vi "Autonomous Independent.vi"() -> ()   [LabVIEW 2016]
doc: "This VI is called when autonomous begins, and will automatically be terminated when autonomous ends. You can carry out timed or sensor driven robot movement independently without needing to return to the caller."
uses:
  <vilib>/Rock Robotics/Network Tables/NT Read Number.vi
  Global 2.vi
  Systems/Global 1.vi
panel:
  out "Present (s)":dbl=3576005670.903064
  out "Time has Elapsed":bool=TRUE
  out "Elapsed Time (s)":dbl=0.26720476150512695
  out "Gyro":dbl=0.23233298402160002
  in  "Oscillate effort":dbl=0.25 format="%#_13g"
  out "Auto Mode":dbl=13.0
  in  "Auton_Modes":T1(array[cluster])=[{"Actions"=[{"Effort"=0.55, "Duration"=3.5, "Action"=enum."Vision Correction", "Encoder"=0.0, "Condition"=FALSE}, {"Effort"=0.0, "Duration"=0.0, "Action"=enum."Nothing", "Encoder"=0.0, "Condition"=FALSE}]}, {"Actions"=[{"Effort"=0.0, "Duration"=0.1, "Action"=enum."Drive Encoder Reset", "Encoder"=0.0, "Condition"=FALSE}, {"Effort"=0.0, "Duration"=0.1, "Action"=enum."Gyro Reset", "Encoder"=0.0, "Condition"=FALSE}, {"Effort"=0.0, "Duration"=4.0, "Action"=enum."Drive", "Encoder"=62.0, "Condition"=FALSE}, {"Effort"=0.15, "Duration"=0.1, "Action"=enum."Turn", "Encoder"=-55.0, "Condition"=FALSE}, {"Effort"=0.0, "Duration"=0.1, "Action"=enum."Gyro Reset", "Encoder"=0.0, "Condition"=FALSE}, {"Effort"=0.0, "Duration"=0.1, "Action"=enum."Drive Encoder Reset", "Encoder"=0.0, "Condition"=FALSE}, {"Effort"=0.0, "Duration"=4.0, "Action"=enum."Drive", "Encoder"=76.0, "Condition"=FALSE}, {"Effort"=1.0, "Duration"=0.25, "Action"=enum."Gear0", "Encoder"=0.0, "Condition"=FALSE}, {"Effort"=0.0, "Duration"=0.1, "Action"=enum."Drive Encoder Reset", "Encoder"=3.0, "Condition"=FALSE}, {"Effort"=0.0, "Duration"=3.0, "Action"=enum."Drive", "Encoder"=-36.0, "Condition"=FALSE}, {"Effort"=0.08, "Duration"=0.0, "Action"=enum."Turn", "Encoder"=15.5, "Condition"=FALSE}, {"Effort"=0.0, "Duration"=0.1, "Action"=enum."Gyro Reset", "Encoder"=0.0, "Condition"=FALSE}, {"Effort"=0.0, "Duration"=0.5, "Action"=enum."Drive Encoder Reset", "Encoder"=0.0, "Condition"=FALSE}, {"Effort"=0.0, "Duration"=5.0, "Action"=enum."Drive", "Encoder"=-94.0, "Condition"=TRUE}]}, {"Actions"=[{"Effort"=0.0, "Duration"=0.1, "Action"=enum."Drive Encoder Reset", "Encoder"=0.0, "Condition"=FALSE}, {"Effort"=0.0, "Duration"=0.1, "Action"=enum."Gyro Reset", "Encoder"=0.0, "Condition"=FALSE}, {"Effort"=0.0, "Duration"=4.0, "Action"=enum."Drive", "Encoder"=76.0, "Condition"=FALSE}, {"Effort"=1.0, "Duration"=0.5, "Action"=enum."Gear0", "Encoder"=0.0, "Condition"=FALSE}, {"Effort"=1.0, "Duration"=0.0, "Action"=enum."Nothing", "Encoder"=0.0, "Condition"=FALSE}, {"Effort"=1.0, "Duration"=0.0, "Action"=enum."Nothing", "Encoder"=0.0, "Condition"=FALSE}, {"Effort"=0.0, "Duration"=0.0, "Action"=enum."Drive Encoder Reset", "Encoder"=0.0, "Condition"=FALSE}, {"Effort"=0.0, "Duration"=0.0, "Action"=enum."Nothing", "Encoder"=0.0, "Condition"=FALSE}, {"Effort"=0.0, "Duration"=0.0, "Action"=enum."Nothing", "Encoder"=0.0, "Condition"=FALSE}, {"Effort"=0.0, "Duration"=10000.0, "Action"=enum."Drive", "Encoder"=-24.0, "Condition"=FALSE}, {"Effort"=0.0, "Duration"=0.0, "Action"=enum."Drive Encoder Reset", "Encoder"=0.0, "Condition"=FALSE}, {"Effort"=-0.4, "Duration"=5.0, "Action"=enum."Nothing", "Encoder"=70.0, "Condition"=FALSE}]}, {"Actions"=[{"Effort"=0.0, "Duration"=0.1, "Action"=enum."Drive Encoder Reset", "Encoder"=6.462, "Condition"=FALSE}, {"Effort"=0.0, "Duration"=0.1, "Action"=enum."Gyro Reset", "Encoder"=0.0, "Condition"=FALSE}, {"Effort"=0.0, "Duration"=1.0, "Action"=enum."Drive", "Encoder"=60.0, "Condition"=FALSE}, {"Effort"=0.15, "Duration"=0.1, "Action"=enum."Turn", "Encoder"=55.0, "Condition"=FALSE}, {"Effort"=0.0, "Duration"=0.1, "Action"=enum."Gyro Reset", "Encoder"=0.0, "Condition"=FALSE}, {"Effort"=-0.25, "Duration"=0.0, "Action"=enum."Drive Encoder Reset", "Encoder"=7.5, "Condition"=FALSE}, {"Effort"=0.0, "Duration"=4.0, "Action"=enum."Drive", "Encoder"=76.0, "Condition"=FALSE}, {"Effort"=1.0, "Duration"=0.25, "Action"=enum."Gear0", "Encoder"=0.0, "Condition"=FALSE}, {"Effort"=0.0, "Duration"=0.1, "Action"=enum."Drive Encoder Reset", "Encoder"=0.0, "Condition"=FALSE}, {"Effort"=0.0, "Duration"=3.0, "Action"=enum."Drive", "Encoder"=-36.0, "Condition"=FALSE}, {"Effort"=0.08, "Duration"=0.0, "Action"=enum."Turn", "Encoder"=-60.0, "Condition"=FALSE}, {"Effort"=0.0, "Duration"=0.1, "Action"=enum."Gyro Reset", "Encoder"=0.0, "Condition"=FALSE}, {"Effort"=0.0, "Duration"=0.5, "Action"=enum."Drive Encoder Reset", "Encoder"=0.0, "Condition"=FALSE}, {"Effort"=0.0, "Duration"=5.0, "Action"=enum."Drive", "Encoder"=30.0, "Condition"=TRUE}]}, {"Actions"=[{"Effort"=0.0, "Duration"=0.1, "Action"=enum."Drive Encoder Reset", "Encoder"=6.462, "Condition"=FALSE}, {"Effort"=0.0, "Duration"=0.1, "Action"=enum."Gyro Reset", "Encoder"=0.0, "Condition"=FALSE}, {"Effort"=0.0, "Duration"=1.0, "Action"=enum."Drive", "Encoder"=60.0, "Condition"=FALSE}, {"Effort"=0.15, "Duration"=0.1, "Action"=enum."Turn", "Encoder"=-55.0, "Condition"=FALSE}, {"Effort"=0.0, "Duration"=0.1, "Action"=enum."Gyro Reset", "Encoder"=0.0, "Condition"=FALSE}, {"Effort"=-0.25, "Duration"=0.0, "Action"=enum."Drive Encoder Reset", "Encoder"=7.5, "Condition"=FALSE}, {"Effort"=0.0, "Duration"=4.0, "Action"=enum."Drive", "Encoder"=76.0, "Condition"=FALSE}, {"Effort"=1.0, "Duration"=0.25, "Action"=enum."Gear0", "Encoder"=0.0, "Condition"=FALSE}, {"Effort"=0.0, "Duration"=0.1, "Action"=enum."Drive Encoder Reset", "Encoder"=0.0, "Condition"=FALSE}, {"Effort"=0.0, "Duration"=3.0, "Action"=enum."Drive", "Encoder"=-36.0, "Condition"=FALSE}, {"Effort"=0.08, "Duration"=0.0, "Action"=enum."Turn", "Encoder"=60.0, "Condition"=FALSE}, {"Effort"=0.0, "Duration"=0.1, "Action"=enum."Gyro Reset", "Encoder"=0.0, "Condition"=FALSE}, {"Effort"=0.0, "Duration"=0.5, "Action"=enum."Drive Encoder Reset", "Encoder"=0.0, "Condition"=FALSE}, {"Effort"=0.0, "Duration"=5.0, "Action"=enum."Drive", "Encoder"=30.0, "Condition"=TRUE}]}, {"Actions"=[{"Effort"=0.0, "Duration"=0.1, "Action"=enum."Drive Encoder Reset", "Encoder"=0.0, "Condition"=FALSE}, {"Effort"=0.0, "Duration"=0.1, "Action"=enum."Gyro Reset", "Encoder"=0.0, "Condition"=FALSE}, {"Effort"=0.0, "Duration"=4.0, "Action"=enum."Drive", "Encoder"=62.0, "Condition"=FALSE}, {"Effort"=0.15, "Duration"=0.1, "Action"=enum."Turn", "Encoder"=55.0, "Condition"=FALSE}, {"Effort"=0.0, "Duration"=0.1, "Action"=enum."Gyro Reset", "Encoder"=0.0, "Condition"=FALSE}, {"Effort"=0.0, "Duration"=0.1, "Action"=enum."Drive Encoder Reset", "Encoder"=0.0, "Condition"=FALSE}, {"Effort"=0.0, "Duration"=4.0, "Action"=enum."Drive", "Encoder"=76.0, "Condition"=FALSE}, {"Effort"=1.0, "Duration"=0.25, "Action"=enum."Gear0", "Encoder"=0.0, "Condition"=FALSE}, {"Effort"=0.0, "Duration"=0.1, "Action"=enum."Drive Encoder Reset", "Encoder"=3.0, "Condition"=FALSE}, {"Effort"=0.0, "Duration"=3.0, "Action"=enum."Drive", "Encoder"=-36.0, "Condition"=FALSE}, {"Effort"=0.08, "Duration"=0.0, "Action"=enum."Turn", "Encoder"=-15.5, "Condition"=FALSE}, {"Effort"=0.0, "Duration"=0.1, "Action"=enum."Gyro Reset", "Encoder"=0.0, "Condition"=FALSE}, {"Effort"=0.0, "Duration"=0.5, "Action"=enum."Drive Encoder Reset", "Encoder"=0.0, "Condition"=FALSE}, {"Effort"=0.0, "Duration"=5.0, "Action"=enum."Drive", "Encoder"=-94.0, "Condition"=TRUE}]}, {"Actions"=[{"Effort"=0.0, "Duration"=0.1, "Action"=enum."Nothing", "Encoder"=0.0, "Condition"=FALSE}, {"Effort"=0.0, "Duration"=0.1, "Action"=enum."Gyro Reset", "Encoder"=0.0, "Condition"=FALSE}, {"Effort"=0.25, "Duration"=5.0, "Action"=enum."Drive", "Encoder"=60000.0, "Condition"=TRUE}, {"Effort"=0.75, "Duration"=1.0, "Action"=enum."Nothing", "Encoder"=0.0, "Condition"=FALSE}, {"Effort"=0.0, "Duration"=1.0, "Action"=enum."Nothing", "Encoder"=0.0, "Condition"=FALSE}, {"Effort"=0.0, "Duration"=0.0, "Action"=enum."Nothing", "Encoder"=0.0, "Condition"=FALSE}]}, {"Actions"=[{"Effort"=0.0, "Duration"=0.1, "Action"=enum."Drive Encoder Reset", "Encoder"=0.0, "Condition"=FALSE}, {"Effort"=0.0, "Duration"=0.1, "Action"=enum."Gyro Reset", "Encoder"=0.0, "Condition"=FALSE}, {"Effort"=0.3, "Duration"=0.0, "Action"=enum."Drive", "Encoder"=24.0, "Condition"=FALSE}, {"Effort"=0.3, "Duration"=3.0, "Action"=enum."Nothing", "Encoder"=0.0, "Condition"=FALSE}, {"Effort"=0.3, "Duration"=2.0, "Action"=enum."Vision Correction", "Encoder"=30.0, "Condition"=FALSE}, {"Effort"=0.2, "Duration"=1.0, "Action"=enum."Drive", "Encoder"=18.5, "Condition"=TRUE}, {"Effort"=1.0, "Duration"=0.0, "Action"=enum."Gear0", "Encoder"=0.0, "Condition"=FALSE}, {"Effort"=-0.2, "Duration"=1.3, "Action"=enum."Drive", "Encoder"=30.0, "Condition"=TRUE}, {"Effort"=0.0, "Duration"=3.0, "Action"=enum."Nothing", "Encoder"=0.0, "Condition"=FALSE}, {"Effort"=0.03, "Duration"=0.0, "Action"=enum."Turn", "Encoder"=0.0, "Condition"=FALSE}, {"Effort"=0.0, "Duration"=0.0, "Action"=enum."Drive", "Encoder"=0.0, "Condition"=FALSE}]}, {"Actions"=[{"Effort"=0.0, "Duration"=0.0, "Action"=enum."Nothing", "Encoder"=0.0, "Condition"=FALSE}]}, {"Actions"=[{"Effort"=0.0, "Duration"=2.5, "Action"=enum."Shoot", "Encoder"=0.0, "Condition"=FALSE}, {"Effort"=0.0, "Duration"=5.0, "Action"=enum."Index", "Encoder"=0.0, "Condition"=FALSE}, {"Effort"=0.25, "Duration"=3.5, "Action"=enum."Nothing", "Encoder"=88.0, "Condition"=FALSE}, {"Effort"=1.0, "Duration"=1.0, "Action"=enum."Nothing", "Encoder"=0.0, "Condition"=FALSE}, {"Effort"=1.0, "Duration"=1.0, "Action"=enum."Nothing", "Encoder"=0.0, "Condition"=FALSE}, {"Effort"=1.0, "Duration"=0.5, "Action"=enum."Nothing", "Encoder"=0.0, "Condition"=FALSE}, {"Effort"=0.0, "Duration"=0.0, "Action"=enum."Nothing", "Encoder"=0.0, "Condition"=FALSE}, {"Effort"=-0.25, "Duration"=0.0, "Action"=enum."Nothing", "Encoder"=3.0, "Condition"=FALSE}, {"Effort"=0.0, "Duration"=0.0, "Action"=enum."Nothing", "Encoder"=0.0, "Condition"=FALSE}, {"Effort"=0.25, "Duration"=0.0, "Action"=enum."Nothing", "Encoder"=24.0, "Condition"=FALSE}, {"Effort"=0.0, "Duration"=0.0, "Action"=enum."Nothing", "Encoder"=0.0, "Condition"=FALSE}, {"Effort"=-0.25, "Duration"=0.0, "Action"=enum."Nothing", "Encoder"=12.0, "Condition"=FALSE}]}, {"Actions"=[{"Effort"=0.0, "Duration"=0.1, "Action"=enum."Drive Encoder Reset", "Encoder"=0.0, "Condition"=FALSE}, {"Effort"=0.0, "Duration"=1.0, "Action"=enum."Gyro Reset", "Encoder"=0.0, "Condition"=FALSE}, {"Effort"=0.3, "Duration"=1.4, "Action"=enum."Drive", "Encoder"=88.0, "Condition"=FALSE}, {"Effort"=0.3, "Duration"=3.0, "Action"=enum."Turn", "Encoder"=2.0, "Condition"=FALSE}, {"Effort"=1.0, "Duration"=1.0, "Action"=enum."Nothing", "Encoder"=0.0, "Condition"=FALSE}, {"Effort"=1.0, "Duration"=1.0, "Action"=enum."Nothing", "Encoder"=0.0, "Condition"=FALSE}, {"Effort"=0.0, "Duration"=0.0, "Action"=enum."Nothing", "Encoder"=0.0, "Condition"=FALSE}, {"Effort"=-0.25, "Duration"=0.0, "Action"=enum."Nothing", "Encoder"=3.0, "Condition"=FALSE}, {"Effort"=0.0, "Duration"=0.0, "Action"=enum."Nothing", "Encoder"=0.0, "Condition"=FALSE}, {"Effort"=0.25, "Duration"=0.0, "Action"=enum."Nothing", "Encoder"=24.0, "Condition"=FALSE}, {"Effort"=0.0, "Duration"=0.0, "Action"=enum."Nothing", "Encoder"=0.0, "Condition"=FALSE}, {"Effort"=-0.25, "Duration"=0.0, "Action"=enum."Nothing", "Encoder"=12.0, "Condition"=FALSE}]}, {"Actions"=[{"Effort"=0.0, "Duration"=1.0, "Action"=enum."Drive Encoder Reset", "Encoder"=0.0, "Condition"=FALSE}, {"Effort"=0.0, "Duration"=1.0, "Action"=enum."Shoot", "Encoder"=0.0, "Condition"=FALSE}, {"Effort"=0.25, "Duration"=5.0, "Action"=enum."Index", "Encoder"=88.0, "Condition"=FALSE}, {"Effort"=1.0, "Duration"=1.0, "Action"=enum."Nothing", "Encoder"=0.0, "Condition"=FALSE}, {"Effort"=1.0, "Duration"=1.0, "Action"=enum."Nothing", "Encoder"=0.0, "Condition"=FALSE}, {"Effort"=1.0, "Duration"=0.5, "Action"=enum."Nothing", "Encoder"=0.0, "Condition"=FALSE}, {"Effort"=0.0, "Duration"=0.0, "Action"=enum."Nothing", "Encoder"=0.0, "Condition"=FALSE}, {"Effort"=-0.25, "Duration"=0.0, "Action"=enum."Nothing", "Encoder"=3.0, "Condition"=FALSE}, {"Effort"=0.0, "Duration"=0.0, "Action"=enum."Nothing", "Encoder"=0.0, "Condition"=FALSE}, {"Effort"=0.25, "Duration"=0.0, "Action"=enum."Nothing", "Encoder"=24.0, "Condition"=FALSE}, {"Effort"=0.0, "Duration"=0.0, "Action"=enum."Nothing", "Encoder"=0.0, "Condition"=FALSE}, {"Effort"=-0.25, "Duration"=0.0, "Action"=enum."Nothing", "Encoder"=12.0, "Condition"=FALSE}]}, {"Actions"=[{"Effort"=0.0, "Duration"=0.1, "Action"=enum."Drive Encoder Reset", "Encoder"=0.0, "Condition"=FALSE}, {"Effort"=0.0, "Duration"=1.0, "Action"=enum."Gyro Reset", "Encoder"=0.0, "Condition"=FALSE}, {"Effort"=0.0, "Duration"=20.0, "Action"=enum."Drive", "Encoder"=60.0, "Condition"=FALSE}, {"Effort"=0.3, "Duration"=4.0, "Action"=enum."Nothing", "Encoder"=0.0, "Condition"=FALSE}, {"Effort"=1.0, "Duration"=1.0, "Action"=enum."Nothing", "Encoder"=0.0, "Condition"=FALSE}, {"Effort"=1.0, "Duration"=0.5, "Action"=enum."Nothing", "Encoder"=0.0, "Condition"=FALSE}, {"Effort"=0.0, "Duration"=0.0, "Action"=enum."Nothing", "Encoder"=0.0, "Condition"=FALSE}, {"Effort"=0.3, "Duration"=0.5, "Action"=enum."Nothing", "Encoder"=24.0, "Condition"=TRUE}, {"Effort"=0.0, "Duration"=0.0, "Action"=enum."Nothing", "Encoder"=0.0, "Condition"=FALSE}, {"Effort"=-0.2, "Duration"=2.0, "Action"=enum."Nothing", "Encoder"=24.0, "Condition"=TRUE}, {"Effort"=0.0, "Duration"=0.0, "Action"=enum."Nothing", "Encoder"=0.0, "Condition"=FALSE}, {"Effort"=-0.25, "Duration"=0.0, "Action"=enum."Nothing", "Encoder"=12.0, "Condition"=FALSE}]}, {"Actions"=[{"Effort"=0.0, "Duration"=0.1, "Action"=enum."Drive Encoder Reset", "Encoder"=0.0, "Condition"=FALSE}, {"Effort"=0.0, "Duration"=0.1, "Action"=enum."Gyro Reset", "Encoder"=0.0, "Condition"=FALSE}, {"Effort"=0.0, "Duration"=4.0, "Action"=enum."Nothing", "Encoder"=4.0, "Condition"=FALSE}, {"Effort"=0.3, "Duration"=0.1, "Action"=enum."Vision Correction", "Encoder"=24.0, "Condition"=FALSE}, {"Effort"=0.0, "Duration"=0.1, "Action"=enum."Nothing", "Encoder"=0.0, "Condition"=FALSE}, {"Effort"=0.3, "Duration"=4.0, "Action"=enum."Nothing", "Encoder"=68.17, "Condition"=FALSE}, {"Effort"=1.0, "Duration"=0.25, "Action"=enum."Nothing", "Encoder"=0.0, "Condition"=FALSE}, {"Effort"=0.0, "Duration"=0.0, "Action"=enum."Nothing", "Encoder"=3.0, "Condition"=FALSE}, {"Effort"=-0.3, "Duration"=3.0, "Action"=enum."Nothing", "Encoder"=36.0, "Condition"=FALSE}, {"Effort"=0.15, "Duration"=0.0, "Action"=enum."Nothing", "Encoder"=31.5, "Condition"=FALSE}, {"Effort"=0.0, "Duration"=0.1, "Action"=enum."Nothing", "Encoder"=0.0, "Condition"=FALSE}]}]
  # "Nothing"
  # "Boiler Right Right side gear"
  # "Middle Gear"
  # "Boiler Right Left Side Gear"
  # "Boiler Left RightSide Gear"
  # "Boiler Left Left Side Gear"
  # "Drive"
  # "Vision Correction"
  # "Hopper"
  # "10 ball"
  # "Farside"
  # "Boilerside-10 ball"
  # "Auto 5"
  # "Auto 6"
  # "Auto 6"
  # "Auto 7"
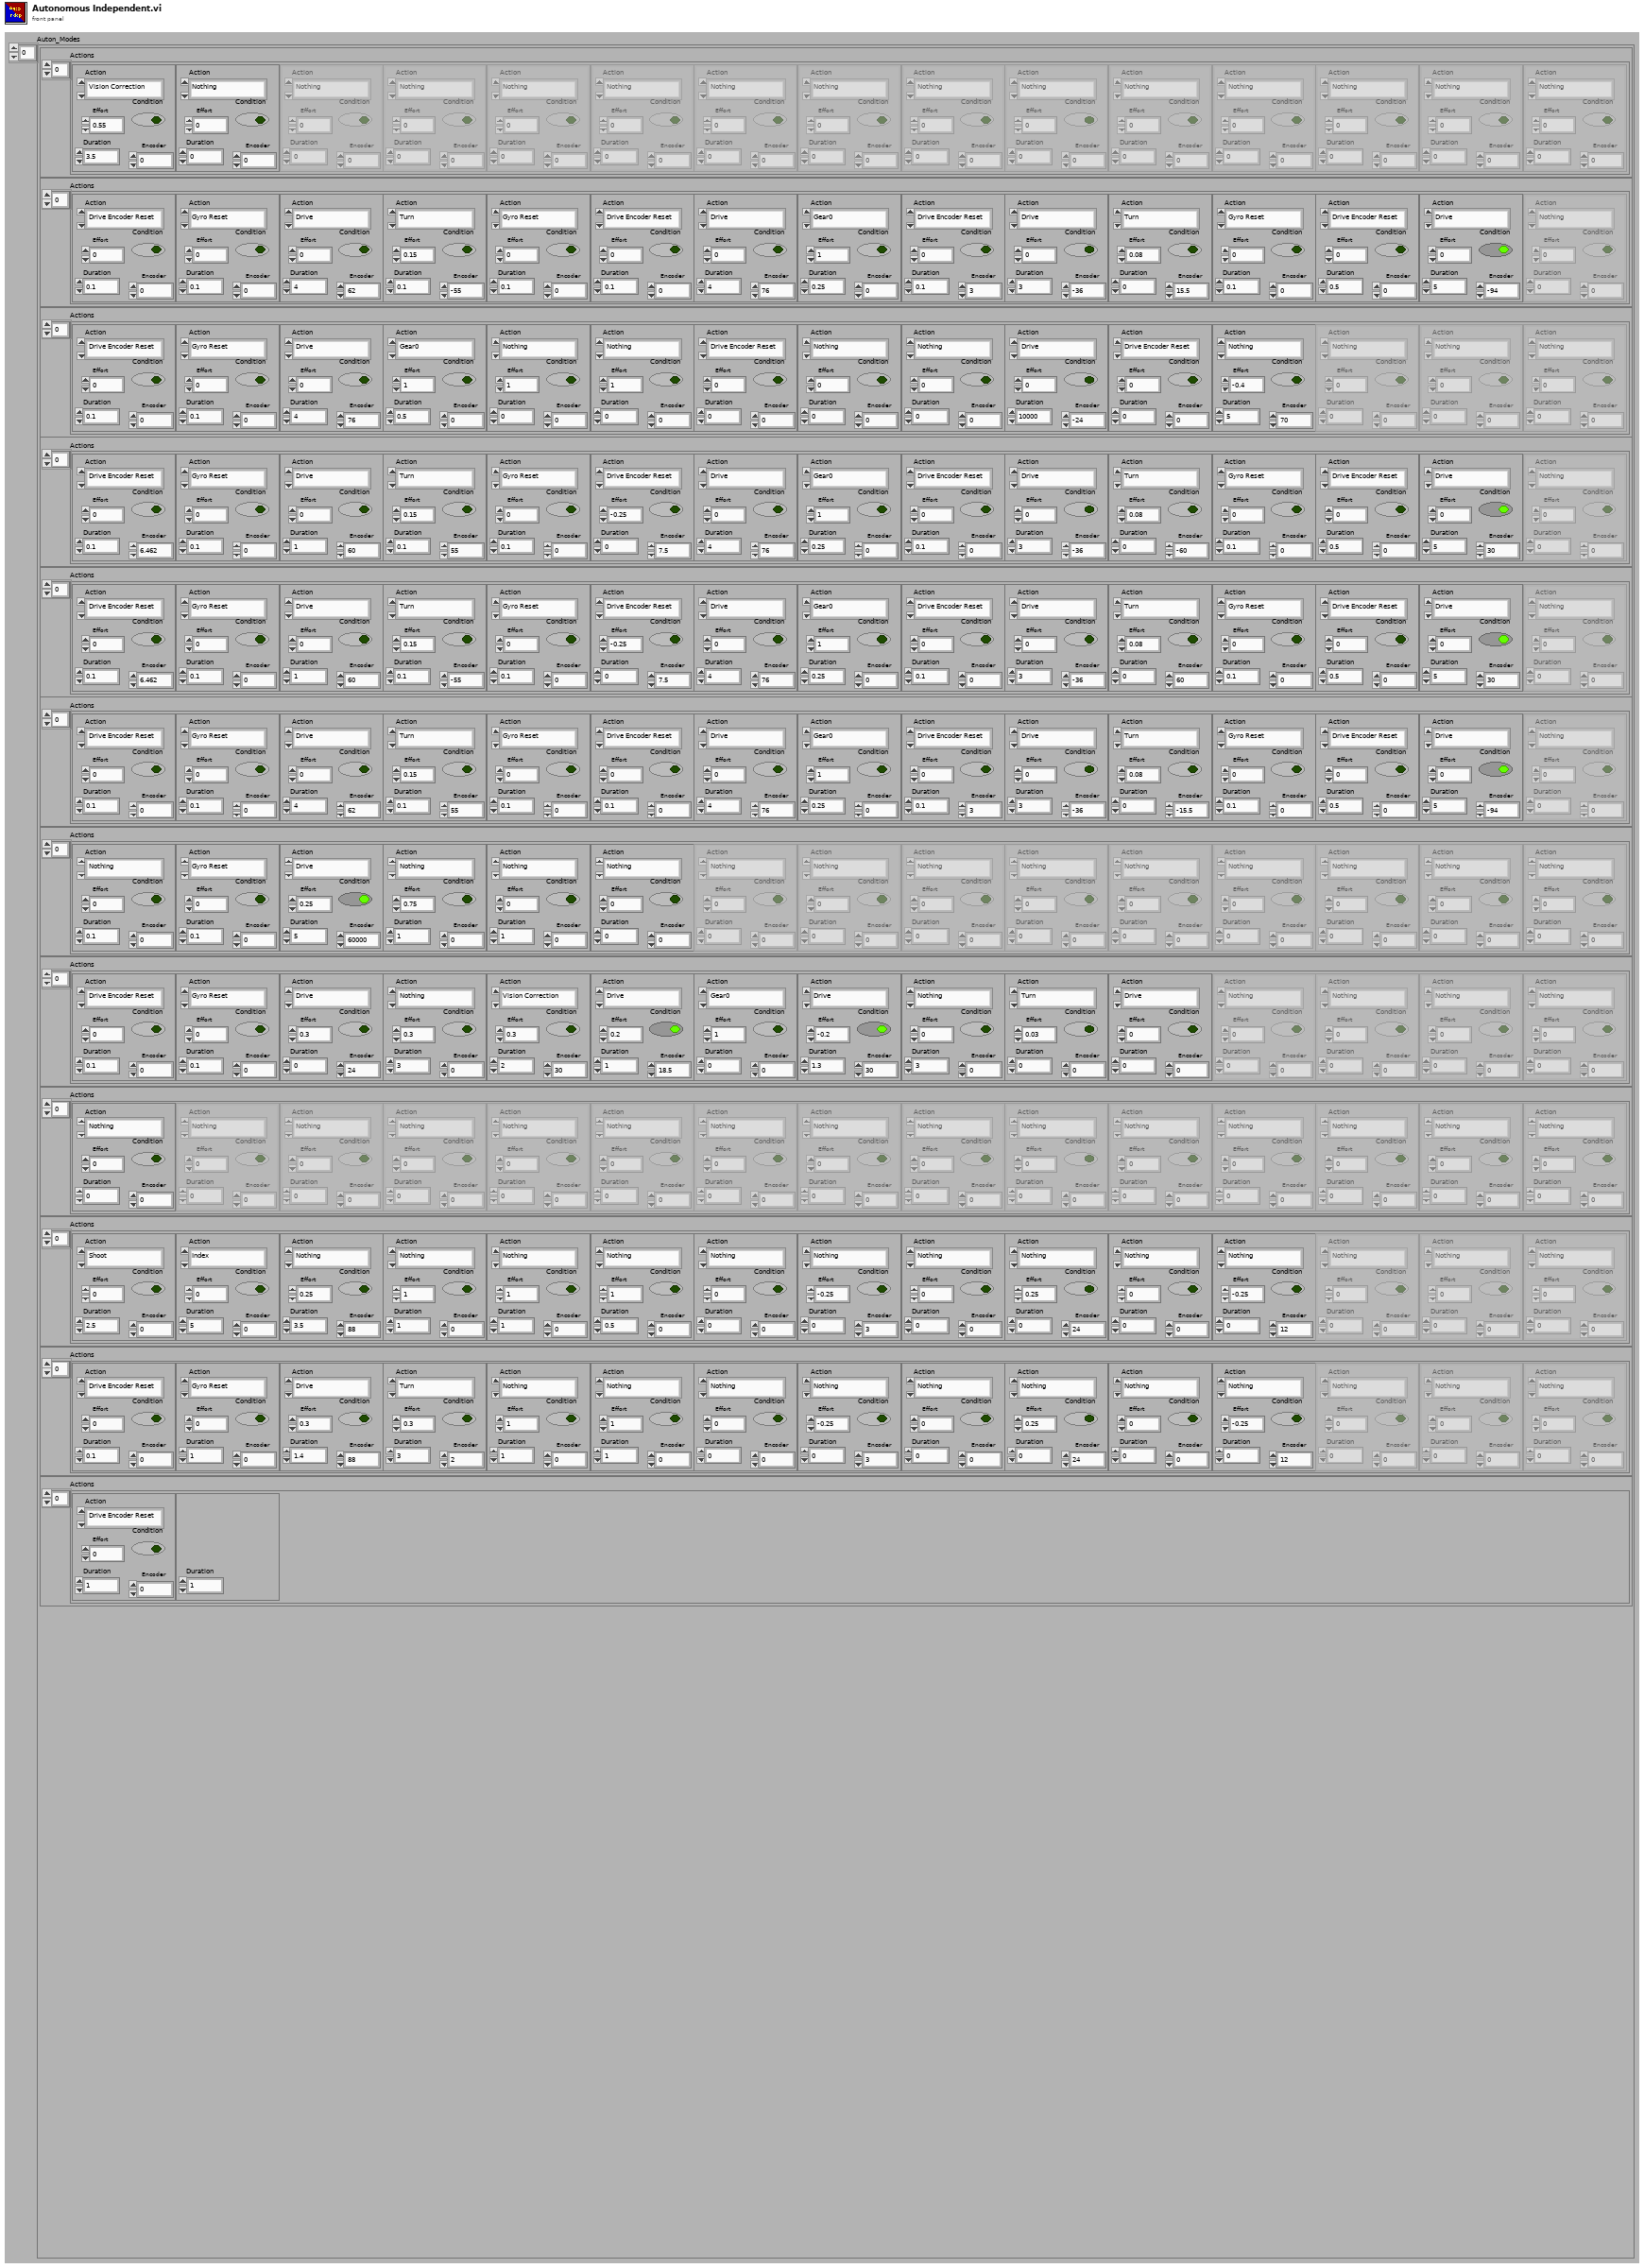
[diagram p1: front panel]
types:
  T1 = cluster{"Actions":cluster{"Effort":dbl, "Duration":dbl, "Action":enum16{"Nothing", "Drive", "Vision Correction", "Turn", "Gear0", "Gear1", "Climb", "Intake", "Index", "Shoot", "Test", "Drive Encoder Reset", "Gyro Reset"}, "Encoder":dbl, "Condition":bool}[]}[]
  T2 = cluster{"Actions":cluster{"Effort":dbl, "Duration":dbl, "Action":enum16{"Nothing", "Drive", "Vision Correction", "Turn", "Gear0", "Gear1", "Climb", "Intake", "Index", "Shoot", "Test", "Drive Encoder Reset", "Gyro Reset"}, "Encoder":dbl, "Condition":bool}[]}
  T3 = cluster{"Effort":dbl, "Duration":dbl, "Action":enum16{"Nothing", "Drive", "Vision Correction", "Turn", "Gear0", "Gear1", "Climb", "Intake", "Index", "Shoot", "Test", "Drive Encoder Reset", "Gyro Reset"}, "Encoder":dbl, "Condition":bool}[]
  T4 = enum16{"Nothing", "Drive", "Vision Correction", "Turn", "Gear0", "Gear1", "Climb", "Intake", "Index", "Shoot", "Test", "Drive Encoder Reset", "Gyro Reset"}
  T5 = typedef "WPI_MotorControlDeviceRef.ctl" = cluster{"DeviceStatus":errorcluster, "Type":T6, "PWM":cluster{"PWM Channel":T7, "DeadBand":T8}, "CAN":cluster{"Device Number":u8, "SetOutput VI Ref":variant, "GetOutput VI Ref":variant, "Enable VI Ref":variant, "Disable VI Ref":variant, "Data":variant}, "Invert":bool}
  T6 = typedef "WPI_MotorControlType.ctl" = enum16{"PWM", "CAN"}
  T7 = typedef "FPGA_DIOPWMChannel.ctl" = enum8{"PWM 0", "PWM 1", "PWM 2", "PWM 3", "PWM 4", "PWM 5", "PWM 6", "PWM 7", "PWM 8", "PWM 9", "PWM MXP 0", "PWM MXP 1", "PWM MXP 2", "PWM MXP 3", "PWM MXP 4", "PWM MXP 5", "PWM MXP 6", "PWM MXP 7", "PWM MXP 8", "PWM MXP 9", "Invalid"}
  T8 = typedef "WPI_PWMDeadband.ctl" = cluster{"Name":string, "maxPositivePwm":i32, "minPositivePwm":i32, "centerPwm":i32, "maxNegativePwm":i32, "minNegativePwm":i32, "angularRange":u16}
  T9 = typedef "WPI_CANTalonSRX_GlobalStatus.ctl" = cluster{"Applied Throttle":dbl, "Module Enabled":bool, "CAN Error":errorcluster, "Closed Loop Error":dbl, "Forward Limit Switch Closed":bool, "Reverse Limit Switch Closed":bool, "Sensor Position":dbl, "Sensor Velocity":dbl, "Current":dbl, "Sticky Fault - Over Temp":bool, "Sticky Fault - Under Voltage":bool, "Sticky Fault - Forward Limit":bool, "Sticky Fault - Reverse Limit":bool, "Sticky Fault - Forward Soft Limit":bool, "Sticky Fault - Reverse Soft Limit":bool, "Brake is Enabled":bool, "Encoder Position":dbl, "Encoder Velocity":dbl, "Encoder Index Count":dbl, "Encoder A Pin State":bool, "Encoder B Pin State":bool, "Encoder Index Pin State":bool, "Analog In":dbl, "Analog In Velocity":dbl, "Temperature (C)":dbl, "Battery Voltage":dbl, "Control 5 Is Supported":bool, "Current Profile Slot Select":dbl, "Pos Div 8":bool, "Vel Div 4":bool, "Pulse Width Position":i32, "Pulse Width Velocity":i32, "Pulse Width Rise To Rise (us)":i32, "Pulse Width Rise To Fall (us)":i32, "Mot Prof Active Is Under Run":bool, "Mot Prof Active Has Under Run":bool, "Mot Prof Active Is Last":bool, "Mot Prof Active Velocity Only":bool, "Mot Prof Active Is Valid":bool, "Mot Prof Buffer Is Full":bool, "Mot Prof Active Profile Slot Select":i32, "Mot Prof NextID":i32, "Mot Prof Count":i32, "Mot Prof Active Velocity":dbl, "Mot Prof Active Position":dbl, "Mot Prof Output Enable":i32}
  T10 = typedef "WPI_GyroDevRef.ctl" = cluster{"DevStatus":errorcluster, "Analog Channel":T11, "Offset":dbl, "Gain (VoltsPerDegree/Second)":dbl, "Gyro Type":enum16{"Analog", "XRS450"}, "Handle":i32, "SPI Bus":T12, "Device Found":bool, "Sample Rate":dbl, "Calibrate On Open":bool}
  T11 = typedef "FPGA_AIChannel.ctl" = enum8{"AI 0", "AI 1", "AI 2", "AI 3", "AI MXP 0", "AI MXP 1", "AI MXP 2", "AI MXP 3", "Invalid"}
  T12 = typedef "spi_bus.ctl" = enum16{"SPI On-Board, CS0", "SPI On-Board, CS1", "SPI On-Board, CS2", "SPI On-Board, CS3", "SPI MXP", "Invalid"}
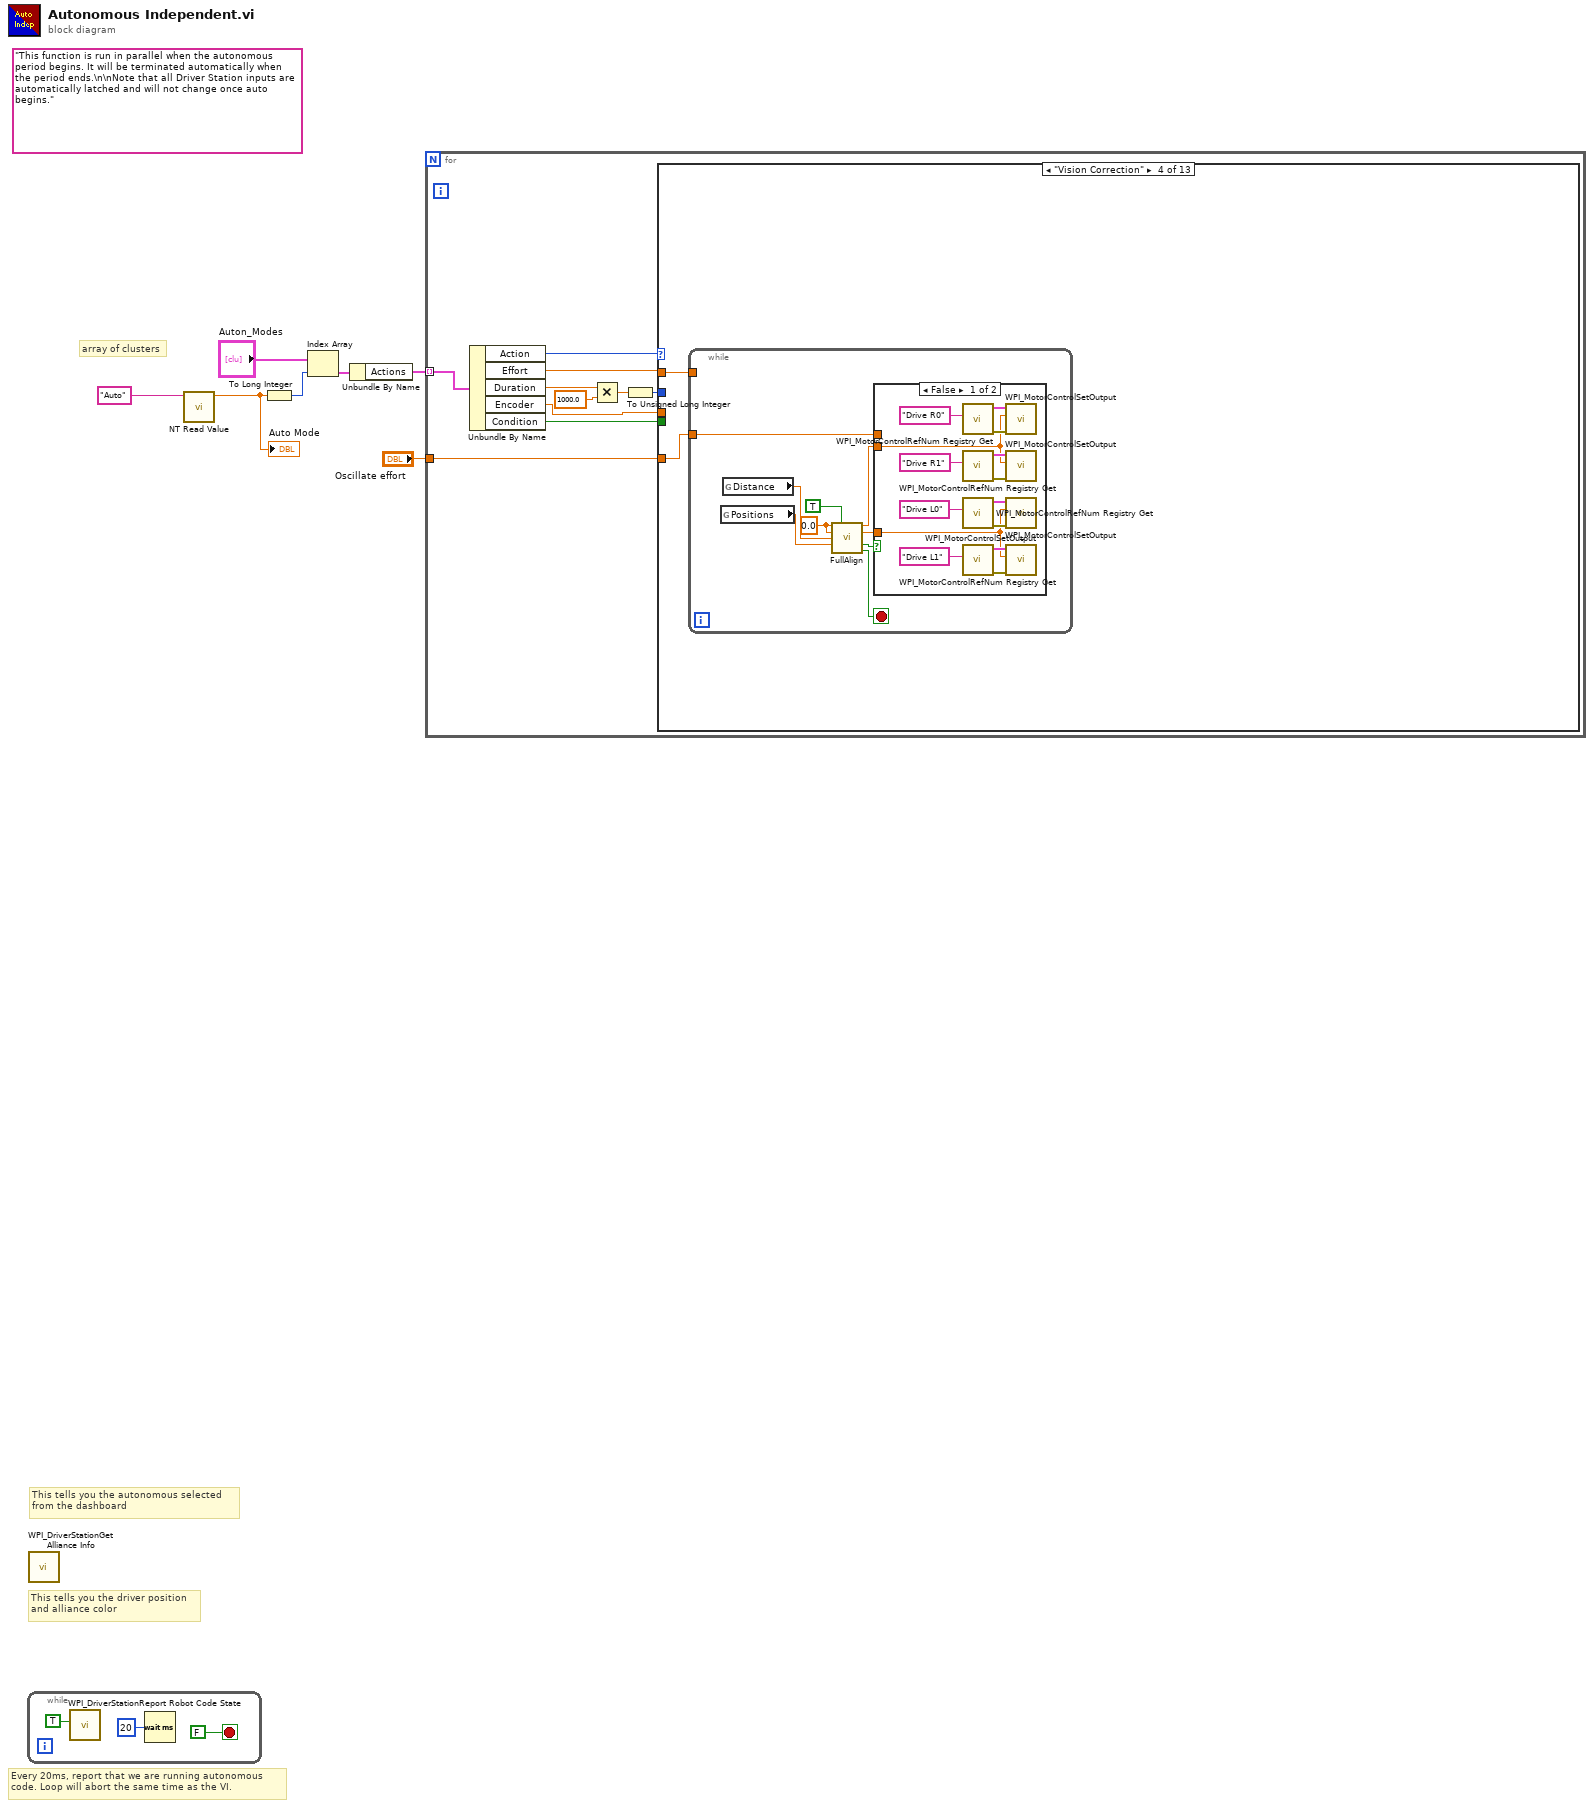
[diagram p0: block diagram]
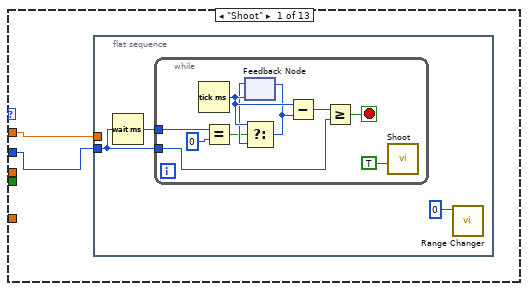
[diagram p2: hidden frame]
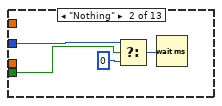
[diagram p3: hidden frame]
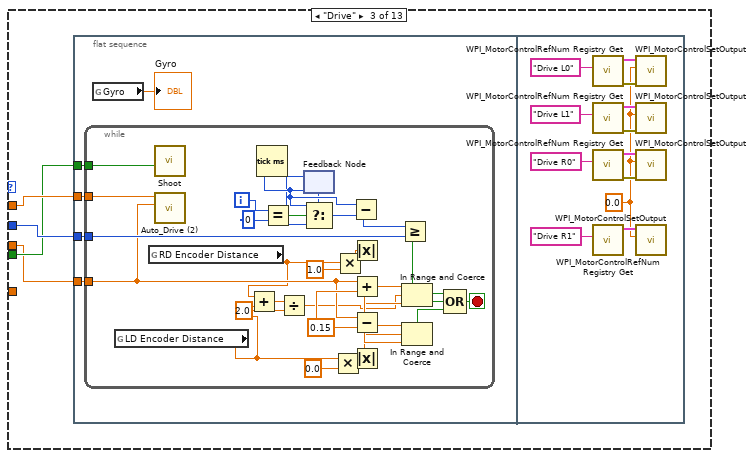
[diagram p4: hidden frame]
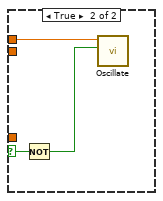
[diagram p5: hidden frame]
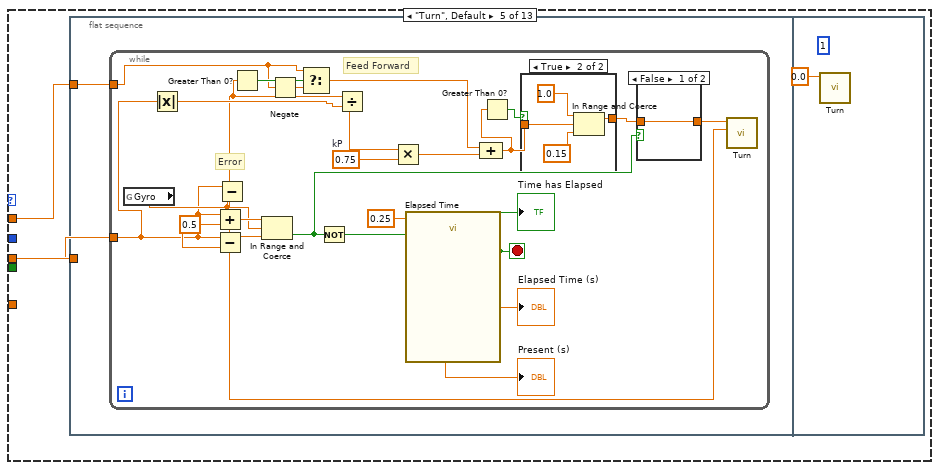
[diagram p6: hidden frame]
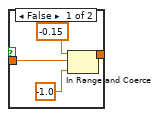
[diagram p7: hidden frame]
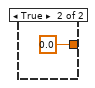
[diagram p8: hidden frame]
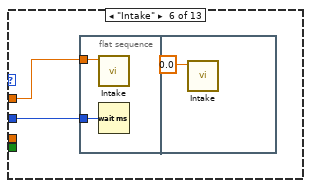
[diagram p9: hidden frame]
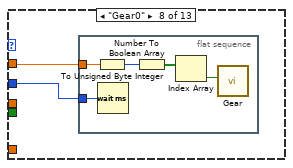
[diagram p11: hidden frame]
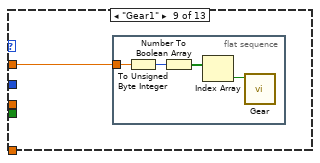
[diagram p12: hidden frame]
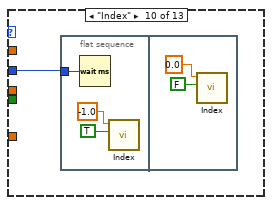
[diagram p13: hidden frame]
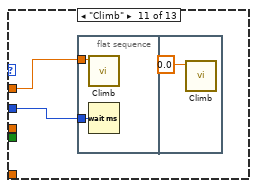
[diagram p14: hidden frame]
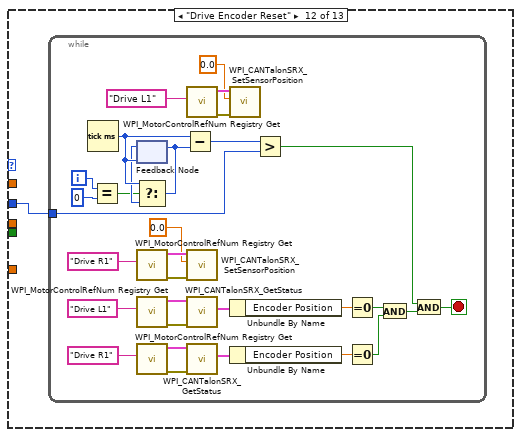
[diagram p15: hidden frame]
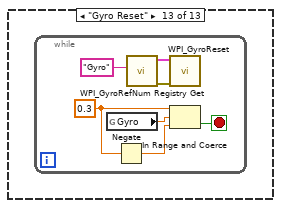
[diagram p16: hidden frame]
diagram:
  (unwired) "This function is run in parallel when the autonomous period begins. It will be terminated automatically when the period ends.\n\nNote that all Driver Station inputs are automatically latched and will not change once auto begins."
  # "This tells you the autonomous selected\nfrom the dashboard"
  # "array of clusters"
  # "Every 20ms, report that we are running autonomous\ncode. Loop will abort the same time as the VI."
  # "This tells you the driver position\nand alliance color"
  n1 = while {
    stop <- FALSE stop-if-true
    n2 = call <vilib>:"WPI_DriverStationReport Robot Code State.vi"("Autonomous"=TRUE) -> ()  [unwired: 10 in, 1 out]
    n3 = Wait (ms)(milliseconds to wait=u32 20) -> ()  [unwired: 1 out]
  }
  n4 = call <vilib>:"WPI_DriverStationGet Alliance Info.vi"() -> ()  [unwired: 12 out]
  n5 = call-poly <vilib>:"NT Read Value.vi"("Name"="Auto") -> ("Numeric"=w2:dbl)  [unwired: 9 in, 1 out]
  "Auto Mode" <- w2
  n6 = To Long Integer(number=w2) -> (32bit integer=w4:i32)
  n7 = Index Array(array="Auton_Modes", index=w4) -> (element=w6:T2)
  n8 = Unbundle By Name(w6) -> ("Actions"=w7:T3)
  n9 = for {
    tunnel: w7 -> [w20] mode=indexing
    tunnel: "Oscillate effort" -> [w12]
    n10 = Unbundle By Name(w20) -> ("Action"=w11:T4, "Effort"=w19:dbl, "Duration"=w18:dbl, "Encoder"=w13:dbl, "Condition"=w15:bool)
    n11 = Multiply(x=w18, y=1000.0) -> (x*y=w17:dbl)
    n12 = To Unsigned Long Integer(number=w17) -> (unsigned 32bit integer=w16:u32)
    n13 = case shown="\"Vision Correction\"" w11 {
      tunnel: w19 -> [w22 _ w43 w90 w118 w157 _ w162 w168 _ w180 _ _]
      tunnel: w16 -> [w21 w38 w42 _ _ w156 _ w161 _ w173 w179 w184 _]
      tunnel: w15 -> [_ w39 w41 _ _ _ _ _ _ _ _ _ _]
      tunnel: w13 -> [_ _ w40 _ w117 _ _ _ _ _ _ _ _]
      tunnel: w12 -> [_ _ _ w89 _ _ _ _ _ _ _ _ _]
      frame "Shoot" {
        n14 = flat-sequence {
          tunnel: w22 -> [_]
          tunnel: w21 -> [w23]
          frame #0 {
            n15 = Wait (ms)(milliseconds to wait=w23) -> (millisecond timer value=w24:u32)
            n16 = while {
              tunnel: w24 -> [w27]
              tunnel: w23 -> [w26]
              stop <- w28 stop-if-true
              n17 = Tick Count (ms)() -> (millisecond timer value=w34:u32)
              n18 = Equal?(x=w27, y=0) -> (x = y?=w32:bool)
              n19 = feedback #1(w34) -> (w33:u32)
              n20 = Select(t=w34, s=w32, f=w33) -> (s? t:f=w30:u32)
              n21 = feedback-in #1(w30) -> ()
              n22 = Subtract(x=w34, y=w30) -> (x-y=w29:u32)
              n23 = Greater Or Equal?(x=w29, y=w26) -> (x >= y?=w28:bool)
              n24 = call "Shoot.vi"("Shoot"=TRUE) -> ()  [unwired: 10 in]
            }
            n25 = call "Range Changer.vi"("POV"=i16 0) -> ()  [unwired: 10 in, 1 out]
          }
        }
      }
      frame "Nothing" {
        n26 = Select(t=w38, s=w39, f=u32 0) -> (s? t:f=w36:u32)
        n27 = Wait (ms)(milliseconds to wait=w36) -> ()  [unwired: 1 out]
      }
      frame "Drive" {
        n28 = flat-sequence {
          tunnel: w43 -> [w48]
          tunnel: w42 -> [w44]
          tunnel: w41 -> [w46]
          tunnel: w40 -> [w47]
          frame #0 {
            n29 = while {
              tunnel: w48 -> [w76]
              tunnel: w47 -> [w58]
              tunnel: w46 -> [w62]
              tunnel: w44 -> [w69]
              i -> [w68]
              stop <- w64 stop-if-true
              w67 = 0.15 ("Range")
              n30 = global read "Global 2.vi" "LD Encoder Distance"() -> (w52:dbl)
              n31 = global read "Global 2.vi" "RD Encoder Distance"() -> (w53:dbl)
              n32 = call "Shoot.vi"("Shoot"=w62) -> ()  [unwired: 10 in]
              n33 = call "Auto_Drive (2).vi"("Target"=w58, "Drive Effort"=w76) -> ()  [unwired: 10 in]
              n34 = Add(x=w53, y=w52) -> (x+y=w51:dbl)
              n35 = Tick Count (ms)() -> (millisecond timer value=w75:u32)
              n36 = Equal?(x=w68, y=0) -> (x = y?=w73:bool)
              n37 = Divide(x=w51, y=2.0) -> (x/y=w49:dbl)
              n38 = feedback #2(w75) -> (w74:u32)
              n39 = Select(t=w75, s=w73, f=w74) -> (s? t:f=w71:u32)
              n40 = feedback-in #2(w71) -> ()
              n41 = Multiply(x=w52, y=0.0) -> (x*y=w56:dbl)
              n42 = Multiply(x=w53, y=1.0) -> (x*y=w57:dbl)
              n43 = Subtract(x=w75, y=w71) -> (x-y=w70:u32)
              n44 = Absolute Value(x=w57) -> ()  [unwired: 1 out]
              n45 = Add(x=w58, y=w67) -> (x+y=w66:dbl)
              n46 = Subtract(x=w58, y=w67) -> (x-y=w65:dbl)
              n47 = Absolute Value(x=w56) -> (abs(x)=w63:dbl)
              n48 = Greater Or Equal?(x=w70, y=w69) -> (x >= y?=w59:bool)
              n49 = In Range and Coerce(upper limit=w66, x=w49, lower limit=w65) -> (In Range?=w60:bool)  [unwired: 1 out]
              n50 = In Range and Coerce(upper limit=w66, x=w63, lower limit=w65) -> (In Range?=w61:bool)  [unwired: 1 out]
              n51 = Compound Arithmetic op=OR(w59, w60, w61) -> (w64:bool)
            }
            n52 = global read "Global 2.vi" "Gyro"() -> (→"Gyro":dbl)
          }
          frame #1 {
            w77 = 0.0 ("Drive L")
            n53 = call <vilib>:"WPI_MotorControlRefNum Registry Get.vi"("refnum name"="Drive L0") -> ("error out"=w83:errorcluster, "MotorControlDevRef"=w84:T5)  [unwired: 9 in]
            n54 = call <vilib>:"WPI_MotorControlRefNum Registry Get.vi"("refnum name"="Drive L1") -> ("error out"=w87:errorcluster, "MotorControlDevRef"=w86:T5)  [unwired: 9 in]
            n55 = call <vilib>:"WPI_MotorControlRefNum Registry Get.vi"("refnum name"="Drive R0") -> ("error out"=w82:errorcluster, "MotorControlDevRef"=w78:T5)  [unwired: 9 in]
            n56 = call <vilib>:"WPI_MotorControlRefNum Registry Get.vi"("refnum name"="Drive R1") -> ("MotorControlDevRef"=w80:T5)  [unwired: 9 in, 1 out]
            n57 = call <vilib>:"WPI_MotorControlSetOutput.vi"("error in (no error)"=w83, "Output"=w77, "MotorControlDevRef"=w84) -> ()  [unwired: 6 in, 3 out]
            n58 = call <vilib>:"WPI_MotorControlSetOutput.vi"("error in (no error)"=w87, "Output"=w77, "MotorControlDevRef"=w86) -> ()  [unwired: 6 in, 3 out]
            n59 = call <vilib>:"WPI_MotorControlSetOutput.vi"("error in (no error)"=w82, "Output"=w77, "MotorControlDevRef"=w78) -> ()  [unwired: 6 in, 3 out]
            n60 = call <vilib>:"WPI_MotorControlSetOutput.vi"("Output"=w77, "MotorControlDevRef"=w80) -> ()  [unwired: 7 in, 3 out]
          }
        }
      }
      frame "Vision Correction" {
        n61 = while {
          tunnel: w90 -> [_]
          tunnel: w89 -> [w93]
          stop <- w94 stop-if-true
          w97 = 0.0
          n62 = global read "Global 1.vi" "Positions"() -> (w95:dbl)
          n63 = global read "Global 1.vi" "Distance"() -> (w96:dbl)
          n64 = call "FullAlign.vi"("Joystick 0"=w97, "Button"=TRUE, "Joystick 1"=w97, "Distance"=w96, "Angle"=w95) -> ("Right Motor"=w99:dbl, "Left Motor"=w98:dbl, "Not In Sight?"=w91:bool, "In Range?"=w94:bool)  [unwired: 7 in]
          n65 = case shown="False" w91 {
            selector: w91 -> [_ w115]
            tunnel: w99 -> [w101 _]
            tunnel: w98 -> [w100 _]
            tunnel: w93 -> [_ w116]
            frame False {
              n66 = call <vilib>:"WPI_MotorControlRefNum Registry Get.vi"("refnum name"="Drive R0") -> ("error out"=w107:errorcluster, "MotorControlDevRef"=w103:T5)  [unwired: 9 in]
              n67 = call <vilib>:"WPI_MotorControlRefNum Registry Get.vi"("refnum name"="Drive R1") -> ("error out"=w102:errorcluster, "MotorControlDevRef"=w105:T5)  [unwired: 9 in]
              n68 = call <vilib>:"WPI_MotorControlRefNum Registry Get.vi"("refnum name"="Drive L0") -> ("error out"=w108:errorcluster, "MotorControlDevRef"=w109:T5)  [unwired: 9 in]
              n69 = call <vilib>:"WPI_MotorControlRefNum Registry Get.vi"("refnum name"="Drive L1") -> ("error out"=w112:errorcluster, "MotorControlDevRef"=w111:T5)  [unwired: 9 in]
              n70 = call <vilib>:"WPI_MotorControlSetOutput.vi"("error in (no error)"=w107, "Output"=w101, "MotorControlDevRef"=w103) -> ()  [unwired: 6 in, 3 out]
              n71 = call <vilib>:"WPI_MotorControlSetOutput.vi"("error in (no error)"=w102, "Output"=w101, "MotorControlDevRef"=w105) -> ()  [unwired: 6 in, 3 out]
              n72 = call <vilib>:"WPI_MotorControlSetOutput.vi"("error in (no error)"=w108, "Output"=w100, "MotorControlDevRef"=w109) -> ()  [unwired: 6 in, 3 out]
              n73 = call <vilib>:"WPI_MotorControlSetOutput.vi"("error in (no error)"=w112, "Output"=w100, "MotorControlDevRef"=w111) -> ()  [unwired: 6 in, 3 out]
            }
            frame True {
              n74 = Not(x=w115) -> (.not. x?=w114:bool)
              n75 = call "Oscillate.vi"("Target In Sight?"=w114, "Effort"=w116) -> ()  [unwired: 10 in]
            }
          }
        }
      }
      frame "Turn", Default {
        n76 = flat-sequence {
          tunnel: w118 -> [w120]
          tunnel: w117 -> [w119]
          frame #0 {
            n77 = while {
              tunnel: w120 -> [w125]
              tunnel: w119 -> [w130]
              stop <- w137 stop-if-true
              w133 = 0.75  # kP
              w144 = 0.5
              # "Feed Forward"
              # "Error"
              n78 = global read "Global 2.vi" "Gyro"() -> (w134:dbl)
              n79 = Absolute Value(x=w130) -> (abs(x)=w129:dbl)
              n80 = Add(x=w130, y=w144) -> (x+y=w143:dbl)
              n81 = Subtract(x=w130, y=w144) -> (x-y=w142:dbl)
              n82 = Subtract(x=w130, y=w134) -> (x-y=w126:dbl)
              n83 = Greater Than 0?(x=w126) -> (x > 0?=w128:bool)
              n84 = In Range and Coerce(upper limit=w143, x=w134, lower limit=w142) -> (In Range?=w136:bool)  [unwired: 1 out]
              n85 = Negate(x=w125) -> (-x=w127:dbl)
              n86 = Select(t=w125, s=w128, f=w127) -> (s? t:f=w124:dbl)
              n87 = Not(x=w136) -> (.not. x?=w138:bool)
              n88 = Divide(x=w126, y=w129) -> (x/y=w131:dbl)
              n89 = Multiply(x=w131, y=w133) -> (x*y=w132:dbl)
              n90 = call "Elapsed Time"("Time Target (s)"=0.25, "Reset"=w138) -> ("Present (s)"=→"Present (s)":dbl, "Elapsed Time (s)"=→"Elapsed Time (s)":dbl, "Time has Elapsed"=w137:bool)  [unwired: 10 in, 5 out]
              "Time has Elapsed" <- w137
              n91 = Compound Arithmetic op=ADD(w124, w132) -> (w121:dbl)
              n92 = Greater Than 0?(x=w121) -> (x > 0?=w122:bool)
              n93 = case shown="True" w122 {
                tunnel: [w145 w150] -> w123
                tunnel: w121 -> [w146 w149]
                frame False {
                  n94 = In Range and Coerce(upper limit=-0.15, x=w146, lower limit=-1.0) -> (coerced(x)=w145:dbl)  [unwired: 1 out]
                }
                frame True {
                  n95 = In Range and Coerce(upper limit=1.0, x=w149, lower limit=0.15) -> (coerced(x)=w150:dbl)  [unwired: 1 out]
                }
              }
              n96 = case shown="False" w136 {
                tunnel: [w153 0.0] -> w135
                tunnel: w123 -> [w153 _]
                frame False {
                }
                frame True {
                }
              }
              n97 = call "Turn.vi"("Gyro"=w126, "Effort"=w135) -> ()  [unwired: 10 in]
            }
          }
          frame #1 {
            (unwired) 1 ("mode")
            n98 = call "Turn.vi"("Effort"=0.0) -> ()  [unwired: 11 in]
          }
        }
      }
      frame "Intake" {
        n99 = flat-sequence {
          tunnel: w157 -> [w159]
          tunnel: w156 -> [w158]
          frame #0 {
            n100 = call "Intake.vi"("Effort"=w159) -> ()  [unwired: 11 in]
            n101 = Wait (ms)(milliseconds to wait=w158) -> ()  [unwired: 1 out]
          }
          frame #1 {
            n102 = call "Intake.vi"("Effort"=0.0) -> ()  [unwired: 11 in]
          }
        }
      }
      frame "Test" {
      }
      frame "Gear0" {
        n103 = flat-sequence {
          tunnel: w162 -> [w167]
          tunnel: w161 -> [w163]
          frame #0 {
            n104 = To Unsigned Byte Integer(number=w167) -> (unsigned 8bit integer=w166:u8)
            n105 = Wait (ms)(milliseconds to wait=w163) -> ()  [unwired: 1 out]
            n106 = Number To Boolean Array(number=w166) -> (Boolean array=w165:bool[])
            n107 = Index Array(array=w165) -> (element=w164:bool)  [unwired: 1 in]
            n108 = call "Gear.vi"("Gear0?"=w164) -> ()  [unwired: 11 in]
          }
        }
      }
      frame "Gear1" {
        n109 = flat-sequence {
          tunnel: w168 -> [w172]
          frame #0 {
            n110 = To Unsigned Byte Integer(number=w172) -> (unsigned 8bit integer=w171:u8)
            n111 = Number To Boolean Array(number=w171) -> (Boolean array=w170:bool[])
            n112 = Index Array(array=w170) -> (element=w169:bool)  [unwired: 1 in]
            n113 = call "Gear.vi"("Gear1?"=w169) -> ()  [unwired: 11 in]
          }
        }
      }
      frame "Index" {
        n114 = flat-sequence {
          tunnel: w173 -> [w174]
          frame #0 {
            n115 = Wait (ms)(milliseconds to wait=w174) -> ()  [unwired: 1 out]
            n116 = call "Index.vi"("Shoot"=TRUE ("Override?"), "Output"=-1.0) -> ()  [unwired: 10 in]
          }
          frame #1 {
            n117 = call "Index.vi"("Shoot"=FALSE ("Override?"), "Output"=0.0) -> ()  [unwired: 10 in]
          }
        }
      }
      frame "Climb" {
        n118 = flat-sequence {
          tunnel: w180 -> [w182]
          tunnel: w179 -> [w181]
          frame #0 {
            n119 = call "Climb.vi"("Effort"=w182) -> ()  [unwired: 11 in]
            n120 = Wait (ms)(milliseconds to wait=w181) -> ()  [unwired: 1 out]
          }
          frame #1 {
            n121 = call "Climb.vi"("Effort"=0.0) -> ()  [unwired: 11 in]
          }
        }
      }
      frame "Drive Encoder Reset" {
        n122 = while {
          tunnel: w184 -> [w187]
          i -> [w189]
          stop <- w185 stop-if-true
          n123 = Tick Count (ms)() -> (millisecond timer value=w195:u32)
          n124 = Equal?(x=w189, y=0) -> (x = y?=w193:bool)
          n125 = feedback #3(w195) -> (w194:u32)
          n126 = Select(t=w195, s=w193, f=w194) -> (s? t:f=w191:u32)
          n127 = feedback-in #3(w191) -> ()
          n128 = call <vilib>:"WPI_MotorControlRefNum Registry Get.vi"("refnum name"="Drive R1") -> ("error out"=w210:errorcluster, "MotorControlDevRef"=w209:T5)  [unwired: 9 in]
          n129 = call <vilib>:"WPI_MotorControlRefNum Registry Get.vi"("refnum name"="Drive L1") -> ("error out"=w205:errorcluster, "MotorControlDevRef"=w200:T5)  [unwired: 9 in]
          n130 = call <vilib>:"WPI_MotorControlRefNum Registry Get.vi"("refnum name"="Drive R1") -> ("error out"=w202:errorcluster, "MotorControlDevRef"=w201:T5)  [unwired: 9 in]
          n131 = Subtract(x=w195, y=w191) -> (x-y=w188:u32)
          n132 = call <vilib>:"WPI_MotorControlRefNum Registry Get.vi"("refnum name"="Drive L1") -> ("error out"=w212:errorcluster, "MotorControlDevRef"=w213:T5)  [unwired: 9 in]
          n133 = call <vilib>:"WPI_CANTalonSRX_SetSensorPosition.vi"("error in (no error)"=w210, "New Sensor Position"=0.0, "CAN Talon SRX Ref"=w209) -> ()  [unwired: 7 in, 2 out]
          n134 = call <vilib>:"WPI_CANTalonSRX_GetStatus.vi"("error in (no error)"=w205, "CAN Talon SRX Ref"=w200) -> ("Talon SRX Status"=w203:T9)  [unwired: 7 in, 2 out]
          n135 = call <vilib>:"WPI_CANTalonSRX_GetStatus.vi"("error in (no error)"=w202, "CAN Talon SRX Ref"=w201) -> ("Talon SRX Status"=w204:T9)  [unwired: 7 in, 2 out]
          n136 = call <vilib>:"WPI_CANTalonSRX_SetSensorPosition.vi"("error in (no error)"=w212, "New Sensor Position"=0.0, "CAN Talon SRX Ref"=w213) -> ()  [unwired: 7 in, 2 out]
          n137 = Unbundle By Name(w203) -> ("Encoder Position"=w198:dbl)
          n138 = Unbundle By Name(w204) -> ("Encoder Position"=w199:dbl)
          n139 = Greater?(x=w188, y=w187) -> (0:w186:bool)
          n140 = Equal To 0?(x=w198) -> (x = 0?=w197:bool)
          n141 = Equal To 0?(x=w199) -> (x = 0?=w196:bool)
          n142 = And(x=w197, y=w196) -> (x .and. y?=w190:bool)
          n143 = And(x=w186, y=w190) -> (x .and. y?=w185:bool)
        }
      }
      frame "Gyro Reset" {
        n144 = while {
          stop <- w216 stop-if-true
          w219 = 0.3
          n145 = global read "Global 2.vi" "Gyro"() -> (w217:dbl)
          n146 = Negate(x=w219) -> (-x=w218:dbl)
          n147 = call <vilib>:"WPI_GyroRefNum Registry Get.vi"("refnum name"="Gyro") -> ("error out"=w221:errorcluster, "GyroDevRef"=w222:T10)  [unwired: 9 in]
          n148 = call <vilib>:"WPI_GyroReset.vi"("error in"=w221, "GyroDevRef"=w222) -> ()  [unwired: 8 in, 2 out]
          n149 = In Range and Coerce(upper limit=w219, x=w217, lower limit=w218) -> (In Range?=w216:bool)  [unwired: 1 out]
        }
      }
    }
  }
